vi "updateZoom.vi"(8 "Zoom old":cluster{"X":sgl, "Y":sgl}, 9 "ratio(h)":bool=TRUE, 10 "update Zoom":bool, 11 "imageRef":refnum<vi>) -> (0 "Zoom out":cluster{"X":sgl, "Y":sgl})   [LabVIEW 2013]
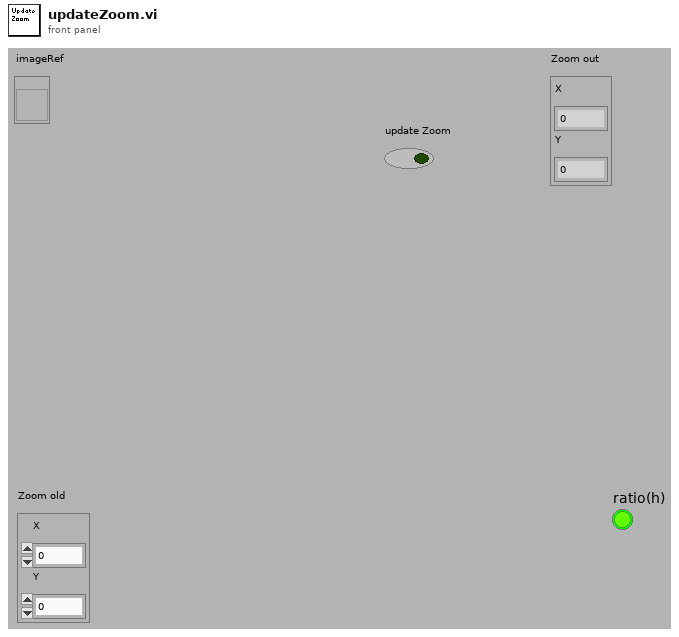
[diagram p1: front panel]
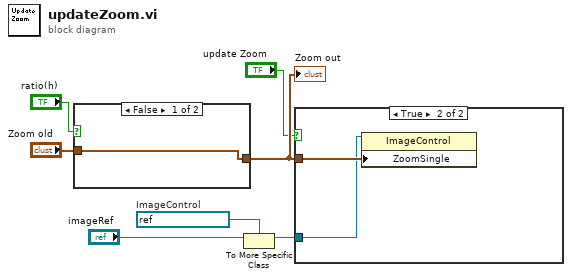
[diagram p0: block diagram]
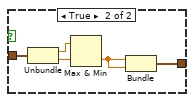
[diagram p2: hidden frame]
diagram:
  w2 = refnum<vi> refnum  # ImageControl
  n1 = case shown="False" "ratio(h)" {
    tunnel: "Zoom old" -> [w8 w11]
    tunnel: [w8 w10] -> w7
    frame False {
    }
    frame True {
      n2 = Unbundle(w11) -> ("X"=w13:sgl, "Y"=w12:sgl)
      n3 = Max & Min(x=w13, y=w12) -> (min(x,y)=w9:sgl)  [unwired: 1 out]
      n4 = Bundle(w9, w9) -> (w10:cluster{sgl, sgl})  [unwired: 1 in]
    }
  }
  "Zoom out" <- w7
  n5 = To More Specific Class(target class=w2, reference="imageRef") -> (specific class reference=w1:refnum<vi>)  [unwired: 1 in, 1 out]
  n6 = case shown="True" "update Zoom" {
    tunnel: w7 -> [_ w15]
    tunnel: w1 -> [_ w14]
    frame False {
    }
    frame True {
      n7 = property class="ImageControl"(reference=w14, "ZoomSingle"=w15) -> ()  [unwired: 1 in, 2 out]
    }
  }
